vi "Read ExposureTime.vi"(8 "error in (no error)":errorcluster, 11 "CCD in":refnum<class "CCD.lvclass">) -> (0 "error out":errorcluster, 2 "ExposureTime [ms]":i32, 3 "CCD out":refnum<class "CCD.lvclass">)   [LabVIEW 2023, in "CCD.lvclass"]
uses:
  CCD.lvclass
  CCD.lvclass/CCD.ctl
  e10f04c6-3c5e-40da-a965-0a1139ef4f67.vi
  Libraries/DeviceManager/DeviceManager.lvlib
  9f7a7c2d-a0c6-4238-a284-e38984d36a8b.vi
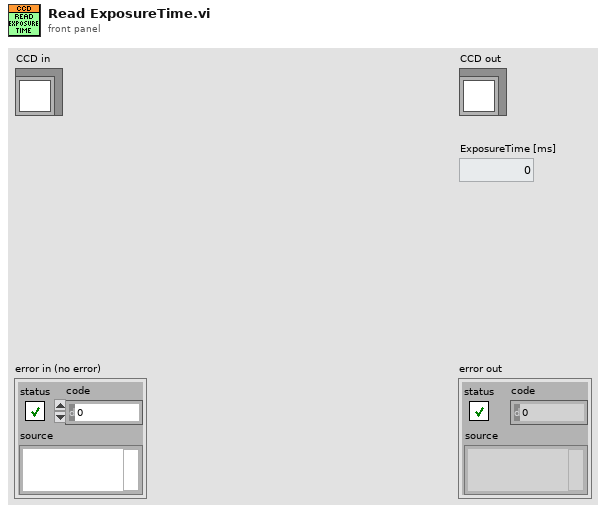
[diagram p1: front panel]
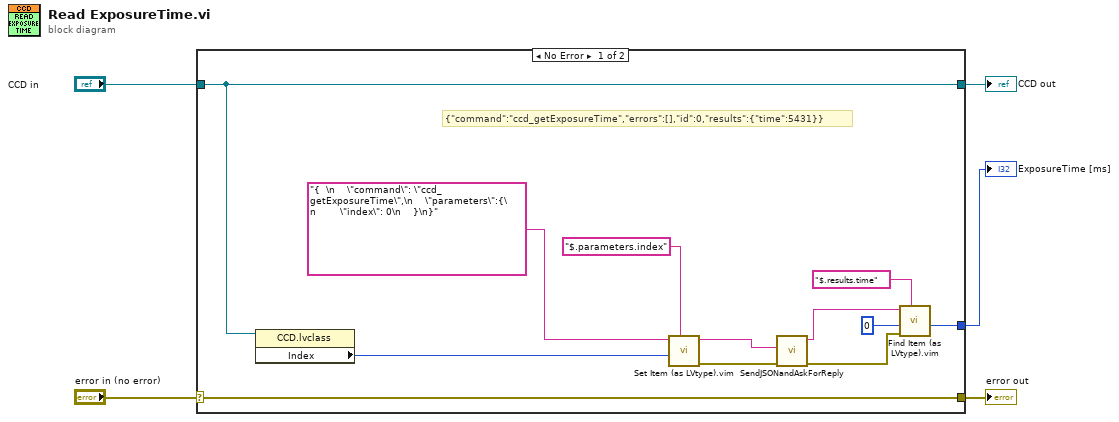
[diagram p0: block diagram]
diagram:
  n1 = case shown="No Error" "error in (no error)" {
    selector: "error in (no error)" -> [w17 w18]
    tunnel: [w17 w18] -> w4
    tunnel: [w11 w19] -> w2
    tunnel: "CCD in" -> [w11 w19]
    tunnel: [w7 _] -> w1
    frame No Error {
      # "{\"command\":\"ccd_getExposureTime\",\"errors\":[],\"id\":0,\"results\":{\"time\":5431}}"
      n2 = property class="CCD.lvclass"(reference=w11) -> ("Index"=w12:i32)  [unwired: 1 in, 2 out]
      n3 = call "Set Item (as LVtype).vim"("$Path or Item Name"="$.parameters.index", "Anything"=w12, "JSON"="{  \n    \"command\": \"ccd_getExposureTime\",\n    \"parameters\":{\n        \"index\": 0\n    }\n}") -> ("error out"=w13:errorcluster, "<JSON>"=w14:string)  [unwired: 5 in, 1 out]
      n4 = call "SendJSONandAskForReply.vi"("error in"=w13, "JSON to be sent"=w14) -> ("error out"=w6:errorcluster, "JSON reply"=w8:string)  [unwired: 7 in, 1 out]
      n5 = call "Find Item (as LVtype).vim"("$Path or Item Name"="$.results.time", "error in (no error)"=w6, "Data Type and Default Value"=0, "JSON"=w8) -> ("Data"=w7:i32)  [unwired: 4 in, 3 out]
    }
    frame Error {
    }
  }
  "error out" <- w4
  "CCD out" <- w2
  "ExposureTime [ms]" <- w1
